vi "OpenConfig.vi"(8 "error in (no error)":errorcluster) -> (0 "error out":errorcluster, 3 "refnum":T1)   [LabVIEW 2017, in "DisplayWindow.lvlib" / "DisplayWindow.lvclass"]
doc: "Opens the DisplayWindow configuration file and provides a refnum."
uses:
  DisplayWindow.lvclass
  <vilib>/Utility/config.llb/Config Data RefNum.ctl
  <vilib>/Utility/config.llb/NI_LVConfig.lvlib
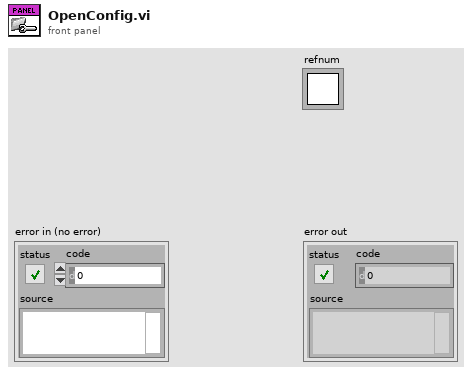
[diagram p1: front panel]
types:
  T1 = typedef "NI_LVConfig.lvlib/Config Data RefNum.ctl" = refnum<k1>
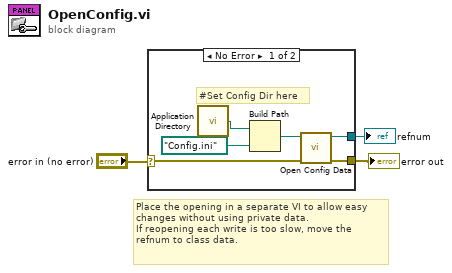
[diagram p0: block diagram]
diagram:
  # "Place the opening in a separate VI to allow easy changes without using private data.\nIf reopening each write is too slow, move the refnum to class data."
  n1 = case shown="No Error" "error in (no error)" {
    selector: "error in (no error)" -> [w4 w10]
    tunnel: [w6 _] -> w1
    tunnel: [w5 w10] -> w2
    frame No Error {
      # "#Set Config Dir here"
      n2 = call <vilib>:"Application Directory.vi"() -> ("Application Directory"=w9:path)
      n3 = Build Path(base path=w9, name or relative path=path "Config.ini") -> (appended path=w7:path)
      n4 = call <vilib>:"Open Config Data.vi"("error in (no error)"=w4, "configuration file path"=w7) -> ("error out"=w5:errorcluster, "refnum"=w6:T1)  [unwired: 7 in, 1 out]
    }
    frame Error {
    }
  }
  "error out" <- w2
  "refnum" <- w1
